vi "XY Graph Are Tool Panels Visible.vi"(8 "Error In":errorcluster, 11 "XY Graph Ref":T2) -> (0 "Error Out":errorcluster, 1 "Any Panel Visible?":bool, 2 "Graph Tool Panels Visibility":T1)   [LabVIEW 2019, in "XY Graph Add-Ons.lvlib"]
uses:
  XY Graph Add-Ons.lvlib
  XY Graph Refnum.ctl
  XY Graph Tool Panels Visibility.ctl
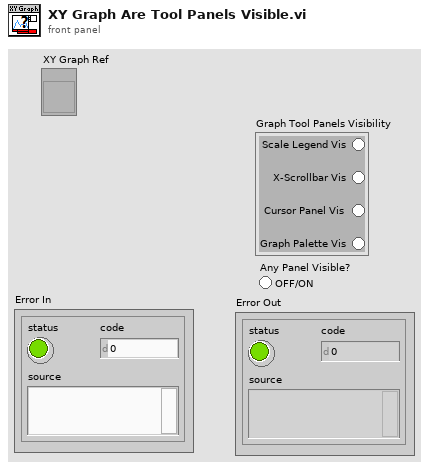
[diagram p1: front panel]
types:
  T1 = typedef "XY Graph Add-Ons.lvlib/XY Graph Tool Panels Visibility.ctl" = cluster{"Scale Legend Vis":bool, "X-Scrollbar Vis":bool, "Cursor Panel Vis":bool, "Graph Palette Vis":bool}
  T2 = typedef "XY Graph Add-Ons.lvlib/XY Graph Refnum.ctl" = refnum<vi>
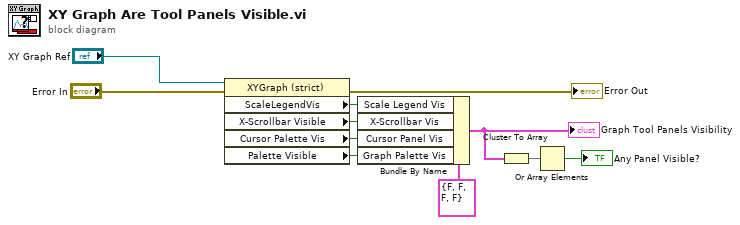
[diagram p0: block diagram]
diagram:
  n1 = property class="XYGraph (strict)"(reference="XY Graph Ref", error in="Error In") -> (error out=→"Error Out":errorcluster, "ScaleLegendVis"=w8:bool, "X-Scrollbar Visible"=w7:bool, "Cursor Palette Vis"=w6:bool, "Palette Visible"=w5:bool)  [unwired: 1 out]
  n2 = Bundle By Name(cluster=T1 {"Scale Legend Vis"=FALSE, "X-Scrollbar Vis"=FALSE, "Cursor Panel Vis"=FALSE, "Graph Palette Vis"=FALSE} ("Graph Tool Panels Visibility"), "Scale Legend Vis"=w8, "X-Scrollbar Vis"=w7, "Cursor Panel Vis"=w6, "Graph Palette Vis"=w5) -> (w3:T1)
  "Graph Tool Panels Visibility" <- w3
  n3 = Cluster To Array(cluster=w3) -> (array=w2:bool[])
  n4 = Or Array Elements(Boolean array=w2) -> (logical OR=→"Any Panel Visible?":bool)
